vi "Get Summary.vi"(7 "Style":enum16{"Diff", "Plain"}(ring), 8 "error in (no error)":errorcluster, 10 "Item":string, 11 "Result Model by Reference In":refnum<class "Result Model by Reference.lvclass">) -> (0 "error out":errorcluster, 2 "Summary":string)   [LabVIEW 2020, in "Result Model by Reference.lvclass"]
uses:
  Result Model by Reference.lvclass
  Result Model by Reference.lvclass/Result Model by Reference.ctl
  Result Model/Result Model.lvclass
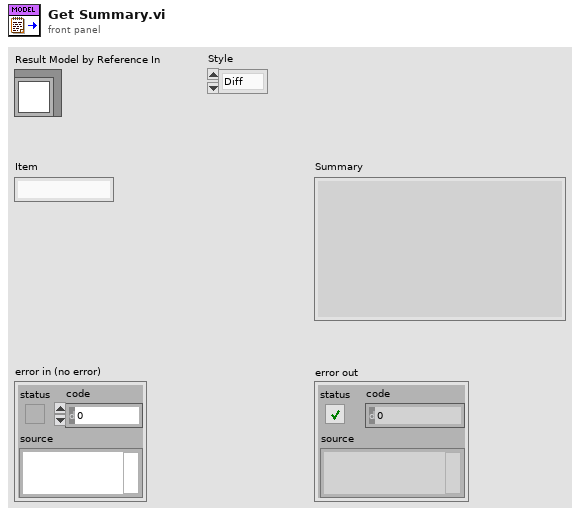
[diagram p1: front panel]
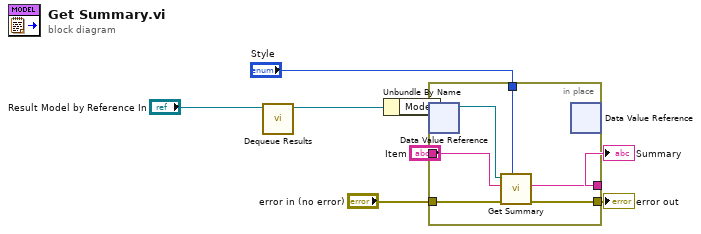
[diagram p0: block diagram]
diagram:
  n1 = call "Dequeue Results.vi"("Result Model by Reference in"="Result Model by Reference In") -> ("Result Model by Reference out"=w2:refnum<class "Result Model by Reference.lvclass">)  [unwired: 10 in]
  n2 = Unbundle By Name(w2) -> ("Model"=w8:refnum<data-value>)
  n3 = in-place {
    in-place-border: "error in (no error)" -> [w14]
    in-place-border: [w13] -> w4
    in-place-border: "Item" -> [w11]
    in-place-border: [w10] -> w3
    in-place-border: "Style" -> [w9]
    n4 = in-place-dvr #1(w8) -> (w12:refnum<class "Result Model.lvclass">)  [unwired: 1 out]
    n5 = call "Get Summary.vi"("Style"=w9, "error in (no error)"=w14, "Item"=w11, "Result Model In"=w12) -> ("error out"=w13:errorcluster, "Summary"=w10:string)  [unwired: 6 in]
    n6 = in-place-dvr #1() -> ()  [unwired: 1 in, 2 out]
  }
  "Summary" <- w3
  "error out" <- w4
